vi "P.AverageSubViSecondMeth.vi"() -> ()   [LabVIEW 2021]
panel:
  in  "array":dbl[](array[numeric])
  out "Average of two arrays":dbl[](array[numeric])
  out "Original array":dbl[](array[numeric])=[6.0, 4.0, 2.0, 1.0]
  out "Array shifted by 1":dbl[](array[numeric])
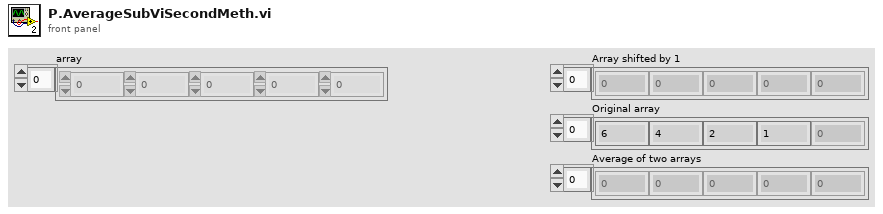
[diagram p1: front panel]
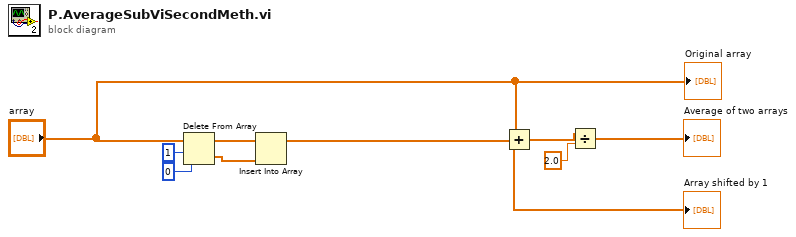
[diagram p0: block diagram]
diagram:
  n1 = Delete From Array "Delete From Array"(array="array", length=1, index=0) -> (deleted portion=w6:dbl[], array with subset deleted=w7:dbl[])
  n2 = Insert Into Array "Insert Into Array"(array=w7, new element=w6) -> (w5:dbl[])  [unwired: 1 in]
  "Array shifted by 1" <- w5
  n3 = Add(x="array", y=w5) -> (x+y=w4:dbl[])
  n4 = Divide(x=w4, y=2.0) -> (x/y=→"Average of two arrays":dbl[])
  "Original array" <- "array"
